vi "query_error_code_database.vi"(10 "code in":i32) -> (1 "code description":string, 2 "code out":i32)   [LabVIEW 2015]
uses:
  is_code_plus_eco.vi
  global_eco.vi
  polys/poly_global_eco_plus.vi
  polys/poly_global_eco_minus.vi
  cores/cores_global_ECO.vi
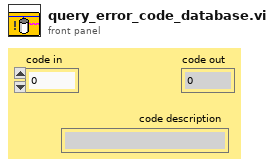
[diagram p1: front panel]
types:
  T1 = enum16{"open", "replace", "create", "open or create", "replace or create", "replace or create with confirmation"}
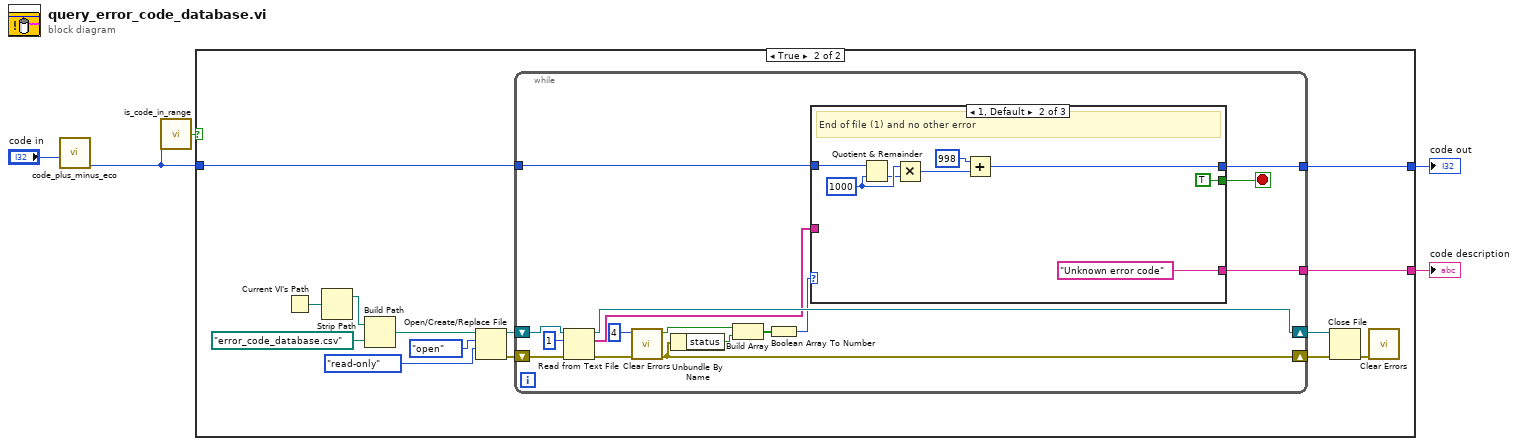
[diagram p0: block diagram]
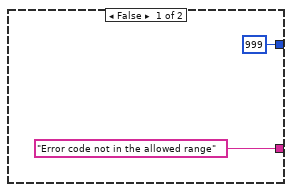
[diagram p2: hidden frame]
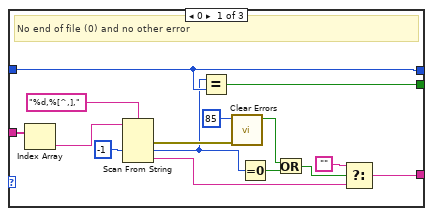
[diagram p3: hidden frame]
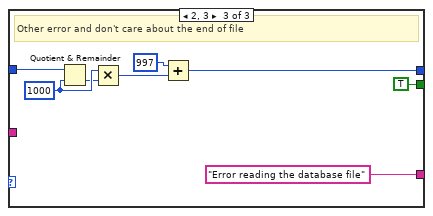
[diagram p4: hidden frame]
diagram:
  n1 = call "code_plus_minus_eco.vi"("code in"="code in") -> ("code w/out ECO"=w1:i32)  [unwired: 9 in, 1 out]
  n2 = call "is_code_in_range.vi"("code (w/out ECO)"=w1) -> ("code in allowed range?"=w2:bool)  [unwired: 4 in]
  n3 = case shown="True" w2 {
    tunnel: w1 -> [_ w11]
    tunnel: ["Error code not in the allowed range" w9] -> w4
    tunnel: [999 ("code w/out ECO") w8] -> w3
    frame False {
    }
    frame True {
      n4 = Current VI's Path() -> (path=w15:path)
      n5 = Strip Path(path=w15) -> (stripped path=w14:path)  [unwired: 1 out]
      n6 = Build Path(base path=w14, name or relative path=path "error_code_database.csv" ("file path")) -> (appended path=w12:path)
      n7 = Open/Create/Replace File(file path (use dialog)=w12, operation (0:open)=T1."open", access (0:read/write)=enum16{"read/write", "read-only", "write-only"}."read-only") -> (refnum out=w21:refnum<file>, error out=w20:errorcluster)  [unwired: 3 in, 1 out]
      n8 = while {
        shift-right: [w36] -> w19
        shift-left: w21 -> [w37]
        tunnel: [w30] -> w9
        shift-right: [w27] -> w18
        shift-left: w20 -> [w35]
        tunnel: [w29] -> w8
        tunnel: w11 -> [w28]
        stop <- w22 stop-if-true
        n9 = Read from Text File(file (use dialog)=w37, count=1, error in=w35) -> (refnum out=w36:refnum<file>, text=w33:string[], error out=w32:errorcluster)  [unwired: 1 in, 1 out]
        n10 = call <vilib>:"Clear Errors.vi"("error in (no error)"=w32, "specific error code to clear (0: all)"=4 ("default value 1")) -> ("error out"=w27:errorcluster, "specific error cleared?"=w23:bool)  [unwired: 4 in]
        n11 = Unbundle By Name(w27) -> ("status"=w26:bool)
        n12 = Build Array(w23, w26) -> (w25:bool[])
        n13 = Boolean Array To Number(Boolean array=w25) -> (number=w24:u32)
        n14 = case shown="1, Default" w24 {
          tunnel: w33 -> [w52 _ _]
          tunnel: [w43 "Unknown error code" "Error reading the database file"] -> w30
          tunnel: [w46 TRUE TRUE] -> w22
          tunnel: [w45 w56 w63] -> w29
          tunnel: w28 -> [w45 w55 w64]
          frame 0 {
            # "No end of file (0) and no other error"
            n15 = Index Array(array=w52) -> (element=w51:string)  [unwired: 1 in]
            n16 = Scan From String(format string="%d,%[^,],", input string=w51, default 1=-1 ("default value 1")) -> (error out=w49:errorcluster, output 1=w44:i32, output 2=w38:string)  [unwired: 3 in, 2 out]
            n17 = Equal?(x=w44, y=w45) -> (x = y?=w46:bool)
            n18 = call <vilib>:"Clear Errors.vi"("error in (no error)"=w49, "specific error code to clear (0: all)"=85) -> ("specific error cleared?"=w42:bool)  [unwired: 4 in, 1 out]
            n19 = Equal To 0?(x=w44) -> (x = 0?=w41:bool)
            n20 = Or(x=w42, y=w41) -> (x .or. y?=w40:bool)
            n21 = Select(t="", s=w40, f=w38) -> (s? t:f=w43:string)
          }
          frame 1, Default {
            w54 = 1000
            # "End of file (1) and no other error"
            n22 = Quotient & Remainder(x=w55, y=w54) -> (floor(x/y)=w53:i32)  [unwired: 1 out]
            n23 = Multiply(x=w54, y=w53) -> (x*y=w58:i32)
            n24 = Add(x=998, y=w58) -> (x+y=w56:i32)
          }
          frame 2, 3 {
            w66 = 1000
            # "Other error and don't care about the end of file"
            n25 = Quotient & Remainder(x=w64, y=w66) -> (floor(x/y)=w65:i32)  [unwired: 1 out]
            n26 = Multiply(x=w66, y=w65) -> (x*y=w68:i32)
            n27 = Add(x=997, y=w68) -> (x+y=w63:i32)
          }
        }
      }
      n28 = Close File(refnum=w19, error in=w18) -> (error out=w10:errorcluster)  [unwired: 1 out]
      n29 = call <vilib>:"Clear Errors.vi"("error in (no error)"=w10) -> ()  [unwired: 5 in, 2 out]
    }
  }
  "code description" <- w4
  "code out" <- w3
